vi "string to filter value.vi"(9 "String":string) -> (10 "Filter Value":T1)   [LabVIEW 2011]
uses:
  filter.ctl
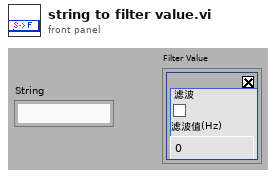
[diagram p1: front panel]
types:
  T1 = typedef "filter.ctl" = cluster{"en":bool, "value":i32, "Boolean":bool}
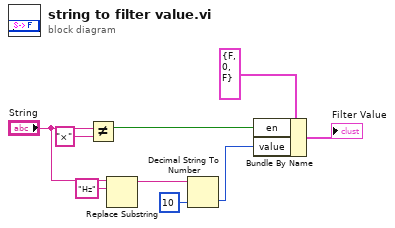
[diagram p0: block diagram]
diagram:
  n1 = Not Equal?(x="String", y="×") -> (x != y?=w6:bool)
  n2 = Replace Substring(4:"Hz" ("substring (\"\")"), 5:"String") -> (1:w3:string)  [unwired: 3 out]
  n3 = Decimal String To Number(string=w3, default (0L)=10 ("default (0 I32)")) -> (number=w2:i32)  [unwired: 2 out]
  n4 = Bundle By Name(cluster=T1 {"en"=FALSE, "value"=0, "Boolean"=FALSE} ("Filter Value"), "en"=w6, "value"=w2) -> (→"Filter Value":T1)
